vi "Get 1D CXT.vi"(5 "format string (%_20f)":string="%_20f", 7 "key description":string, 8 "sections":string[](array[string]), 9 "numeric":cxt[](array[numeric]), 11 "info data":string) -> (0 "sections out":string[](array[string]), 1 "key found?":bool, 2 "value":cxt[](array[numeric]) format="%.2f", 3 "info data out":string)   [LabVIEW 2013, in "infolib.lvlib"]
doc: "Add a new numeric key to Info Data string. If section exists in Info Data string, inserts key into this section."
uses:
  infolib.lvlib
  Get 2D CXT.vi
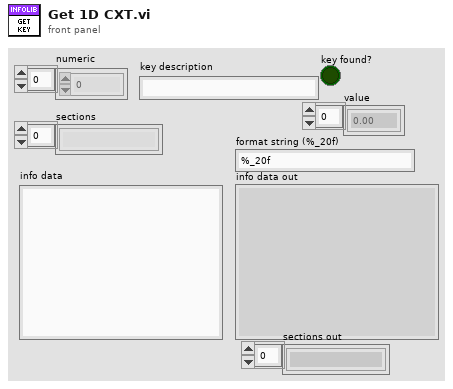
[diagram p1: front panel]
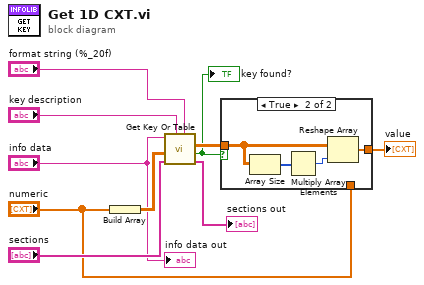
[diagram p0: block diagram]
diagram:
  n1 = Build Array("numeric") -> (w10:cxt[][])
  n2 = call-poly "Get Key Or Table.vi"("format string (%_20f)"="format string (%_20f)", "key description"="key description", "sections"="sections", "numeric"=w10, "info data"="info data") -> ("sections out"=→"sections out":string[], "key found?"=w2:bool, "value"=w4:cxt[][])  [unwired: 3 in, 1 out]
  "key found?" <- w2
  n3 = case shown="True" w2 {
    tunnel: w4 -> [_ w13]
    tunnel: [w11 w12] -> w3
    tunnel: "numeric" -> [w11 _]
    frame False {
    }
    frame True {
      n4 = Array Size(array=w13) -> (size(s)=w14:i32[])
      n5 = Multiply Array Elements(1:w14) -> (0:w15:i32)
      n6 = Reshape Array(w13, w15) -> (w12:cxt[])
    }
  }
  "value" <- w3
  "info data out" <- "info data"
